vi "DEMO.vi"() -> ()   [LabVIEW 2013]
uses:
  VI/DBL Constant.vi
  VI/Integer Constant.vi
  VI/String Constant.vi
  Resource Constant.lvlib
panel:
  out "发动机温度":string
  out "LPT Address":i32 format="%.0x"
  out "PI":dbl
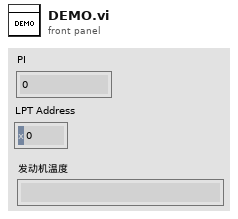
[diagram p1: front panel]
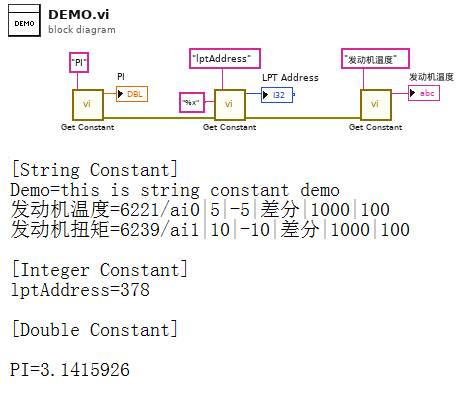
[diagram p0: block diagram]
diagram:
  n1 = call-poly "Get Constant.vi"("Name"="PI") -> ("error out"=w7:errorcluster, "Value"=→"PI":dbl)  [unwired: 9 in]
  n2 = call-poly "Get Constant.vi"("error in (no error)"=w7, "格式字符串"="%x", "Name"="lptAddress") -> ("error out"=w3:errorcluster, "Value"=→"LPT Address":i32)  [unwired: 7 in]
  n3 = call-poly "Get Constant.vi"("error in (no error)"=w3, "Name"="发动机温度") -> ("Value"=→"发动机温度":string)  [unwired: 8 in, 1 out]
